vi "replaceNodeValue.vi"(7 "searchInElement":string, 8 "error in (no error)":errorcluster, 9 "replaceWith":string, 10 "replaceElement":string, 11 "xmlNode in":refnum<class "xmlNode.lvclass">) -> (0 "error out":errorcluster, 2 "xmlNodeReplacement":refnum<class "xmlNode.lvclass">, 3 "xmlNode out":refnum<class "xmlNode.lvclass">)   [LabVIEW 2009, in "Tools.lvlib" / "xml.lvlib" / "xmlNode.lvclass"]
uses:
  xmlNode.lvclass
  XmlParser.lvclass
panel:
  out "String":string
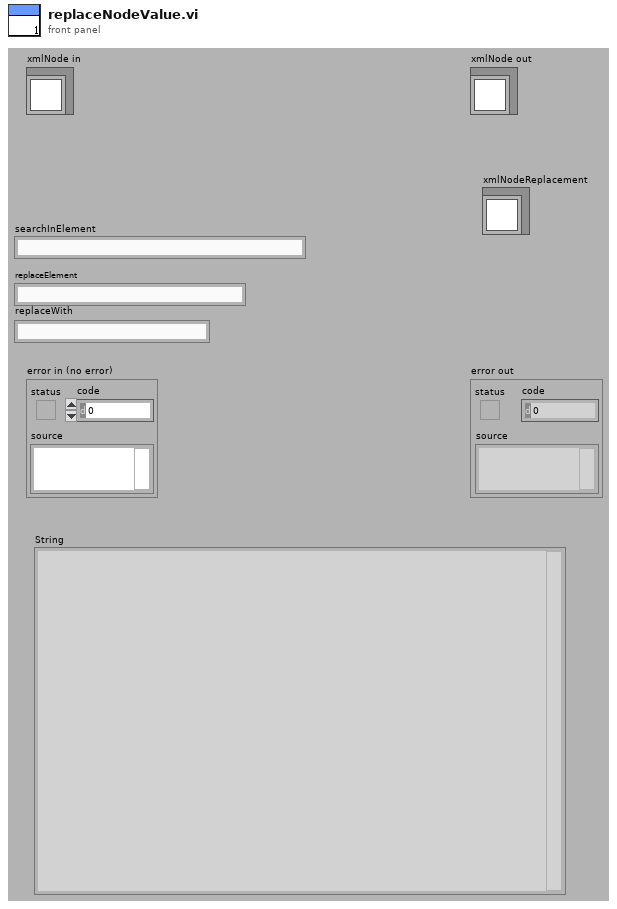
[diagram p1: front panel]
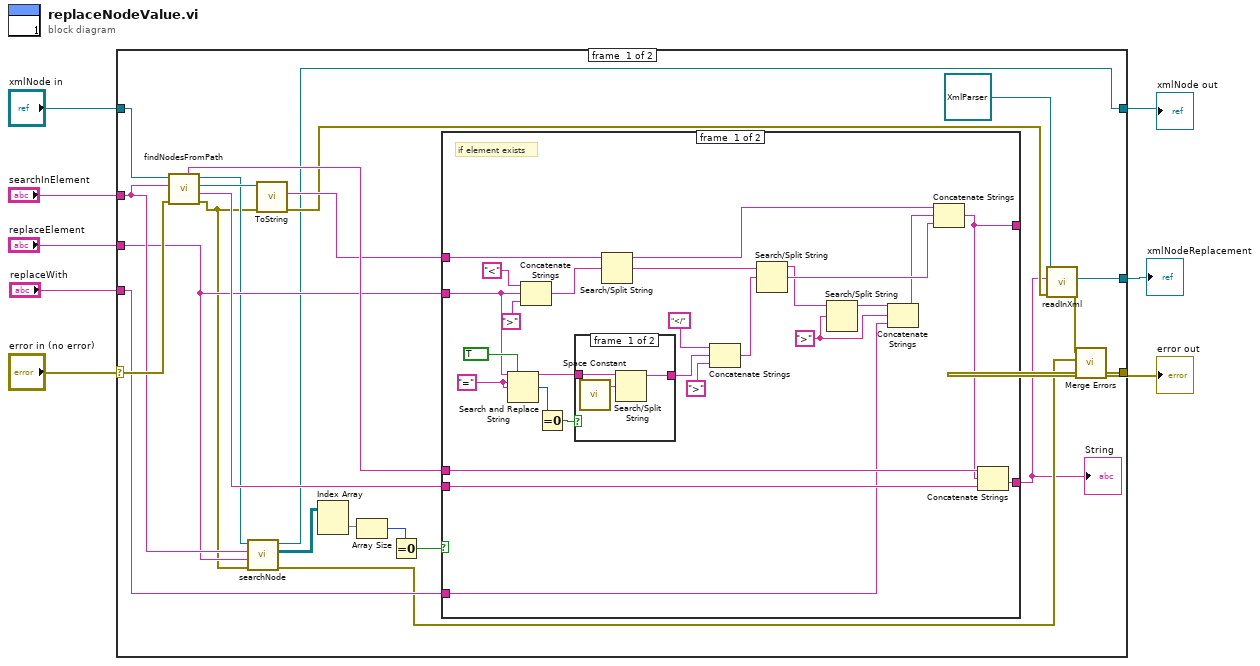
[diagram p0: block diagram]
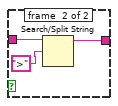
[diagram p2: hidden frame]
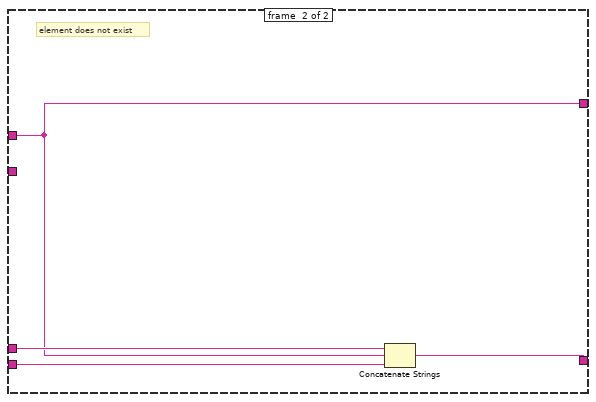
[diagram p3: hidden frame]
diagram:
  n1 = case shown="No Error" "error in (no error)" {
    selector: "error in (no error)" -> [w30 w69]
    tunnel: [w12 w69] -> w7
    tunnel: [w10 w68] -> w5
    tunnel: "xmlNode in" -> [w21 w68]
    tunnel: "searchInElement" -> [w20 _]
    tunnel: "replaceElement" -> [w19 _]
    tunnel: "replaceWith" -> [w22 _]
    tunnel: [w11 _] -> w1
    frame #0 {
      n2 = call "findNodesFromPath.vi"("error in (no error)"=w30, "searchInElement"=w20, "xmlNode in"=w21) -> ("error out"=w15:errorcluster, "rest of xml"=w27:string, "xmlNode"=w29:refnum<class "xmlNode.lvclass">, "xmlNode out"=w18:refnum<class "xmlNode.lvclass">, "xml before"=w28:string)  [unwired: 4 in]
      n3 = call-dynamic "searchNode.vi"("error in (no error)"=w15, "searchElementName"=w19, "searchElementIn"=w20, "xmlNode in"=w18) -> ("error out"=w13:errorcluster, "arrayXmlNodes"=w16:refnum<class "xmlNode.lvclass">[][], "xmlNode out"=w10:refnum<class "xmlNode.lvclass">)  [unwired: 5 in]
      n4 = call-dynamic "ToString.vi"("error in (no error)"=w15, "xmlNode in"=w29) -> ("error out"=w23:errorcluster, "xml"=w26:string)  [unwired: 7 in, 1 out]
      n5 = Index Array(array=w16) -> (element=w17:refnum<class "xmlNode.lvclass">[])  [unwired: 2 in]
      n6 = Array Size(array=w17) -> (size(s)=w31:i32)
      n7 = Equal To 0?(x=w31) -> (x = 0?=w25:bool)
      n8 = case shown="True" w25 {
        tunnel: w28 -> [w57 w67]
        tunnel: w27 -> [w56 w66]
        tunnel: w26 -> [w37 w64]
        tunnel: w19 -> [w36 _]
        tunnel: [w35 w64] -> _
        tunnel: [w34 w65] -> w9
        tunnel: w22 -> [w33 _]
        frame #0 {
          w38 = ">"
          w52 = "="
          # "if element exists"
          n9 = Search and Replace String(replace all?=TRUE, input string=w36, search string=w52, replace string=w52) -> (result string=w49:string, number of replacements=w51:i32)  [unwired: 4 in, 2 out]
          n10 = Concatenate Strings("<", w36, ">") -> (w54:string)
          n11 = Equal To 0?(x=w51) -> (x = 0?=w50:bool)
          n12 = case shown="True" w50 {
            tunnel: w49 -> [w60 w63]
            tunnel: [w58 w61] -> w46
            frame #0 {
              n13 = call <vilib>:"Space Constant.vi"() -> ("String"=w59:string)
              n14 = Search/Split String(string=w60, search string/char (-)=w59) -> (substring before match=w58:string)  [unwired: 1 in, 2 out]
            }
            frame #1 {
              n15 = Search/Split String(string=w63, search string/char (-)=">") -> (substring before match=w61:string)  [unwired: 1 in, 2 out]
            }
          }
          n16 = Search/Split String(string=w37, search string/char (-)=w54) -> (substring before match=w53:string, match + rest of string=w42:string)  [unwired: 1 in, 1 out]
          n17 = Concatenate Strings("</", w46, ">") -> (w44:string)
          n18 = Search/Split String(string=w42, search string/char (-)=w44) -> (substring before match=w41:string, match + rest of string=w43:string)  [unwired: 1 in, 1 out]
          n19 = Search/Split String(string=w41, search string/char (-)=w38) -> (substring before match=w40:string)  [unwired: 1 in, 2 out]
          n20 = Concatenate Strings(w40, w38, w33) -> (w39:string)
          n21 = Concatenate Strings(w53, w39, w43) -> (w35:string)
          n22 = Concatenate Strings(w57, w35, w56) -> (w34:string)
        }
        frame #1 {
          # "element does not exist"
          n23 = Concatenate Strings(w67, w64, w66) -> (w65:string)
        }
      }
      "String" <- w9
      n24 = call "readInXml.vi"("error in (no error)"=w23, "xmlString"=w9, "XmlParser in"=refnum<class "XmlParser.lvclass"> refnum ("Tools.lvlib:xml.lvlib:XmlParser.lvclass")) -> ("error out"=w14:errorcluster, "xmlNode"=w11:refnum<class "xmlNode.lvclass">)  [unwired: 6 in, 1 out]
      n25 = call <vilib>:"Merge Errors.vi"("error in 2 (no error)"=w13, "error in 1 (no error)"=w14) -> ("error out"=w12:errorcluster)  [unwired: 5 in]
    }
    frame #1 {
    }
  }
  "error out" <- w7
  "xmlNode out" <- w5
  "xmlNodeReplacement" <- w1
